vi "LaunchNewActivity.vi"(8 "error in (no error)":errorcluster, 10 "New Activity":refnum<class "SMO.Activity.lvclass">, 11 "SMO.Activity in":refnum<class "SMO.Activity.lvclass">) -> (0 "error out":errorcluster, 3 "SMO.Activity out":refnum<class "SMO.Activity.lvclass">)   [LabVIEW 2015, in "SMO.Activity.lvclass"]
uses:
  SMO.Activity.lvclass
  <vilib>/JKI/JKI SMO/SMO/SMO.lvclass
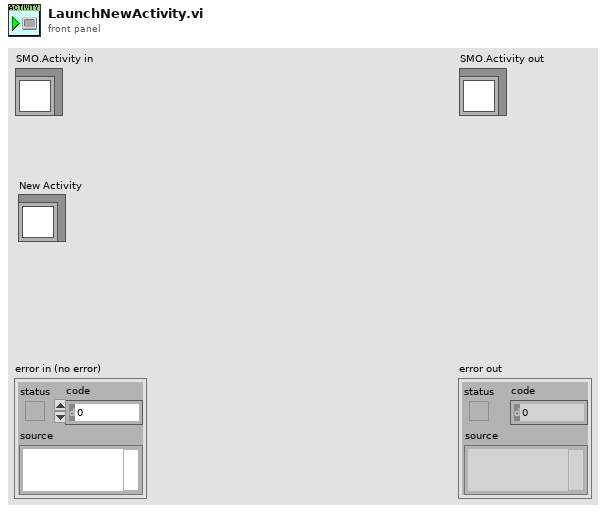
[diagram p1: front panel]
types:
  T1 = typedef "SMO.lvclass/SMOState --Enum.ctl" = enum16{"unknown", "Created", "Started", "Stopped"}
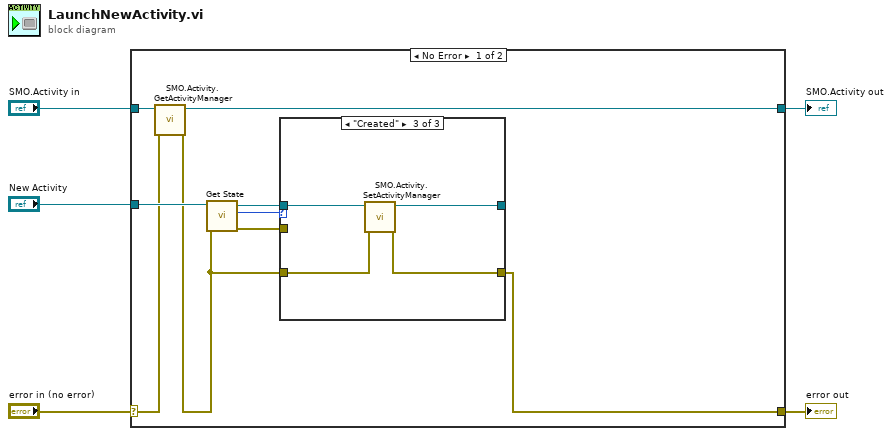
[diagram p0: block diagram]
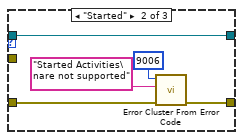
[diagram p3: hidden frame]
diagram:
  n1 = case shown="No Error" "error in (no error)" {
    selector: "error in (no error)" -> [w9 w27]
    tunnel: [w6 w27] -> w4
    tunnel: [w10 w26] -> w2
    tunnel: "SMO.Activity in" -> [w11 w26]
    tunnel: "New Activity" -> [w14 _]
    frame No Error {
      n2 = call "SMO.Activity.GetActivityManager.vi"("error in (no error)"=w9, "SMO.Activity"=w11) -> ("error out"=w7:errorcluster, "SMO.Activity out"=w10:refnum<class "SMO.Activity.lvclass">)  [unwired: 8 in]
      n3 = call <vilib>:"Get State.vi"("error in (no error)"=w7, "SMO"=w14) -> ("error out"=w12:errorcluster, "SMO State"=w13:T1, "SMO out"=w8:refnum<class "SMO.Activity.lvclass">)  [unwired: 7 in]
      n4 = case shown="\"Created\"" w13 {
        tunnel: w12 -> [_ _ _]
        tunnel: w8 -> [w15 w17 w25]
        tunnel: w7 -> [w16 w21 w24]
        tunnel: [w16 w20 w23] -> w6
        tunnel: [w15 w17 w22] -> _
        frame "unknown", Default {
        }
        frame "Started" {
          n5 = call <vilib>:"Error Cluster From Error Code.vi"("error in (no error)"=w21, "error message (\"\")"="Started Activities\nare not supported" ("error message (\"\")"), "error code (0)"=9006) -> ("error out"=w20:errorcluster)  [unwired: 6 in]
        }
        frame "Created" {
          n6 = call "SMO.Activity.SetActivityManager.vi"("error in (no error)"=w24, "SMO.Activity in"=w25) -> ("error out"=w23:errorcluster, "SMO.Activity out"=w22:refnum<class "SMO.Activity.lvclass">)  [unwired: 8 in]
        }
      }
    }
    frame Error {
    }
  }
  "error out" <- w4
  "SMO.Activity out" <- w2
